vi "ANAL_DeriveData.vi"(10 "GUI Cluster":T1, 11 "Main Data Array":T2 {"Run Data Cluster"."Temperature B" scale=0.0..100.0; "Run Data Cluster"."Temperature A" scale=0.0..100.0}) -> (2 "GUI Cluster Out":T1, 3 "Main Data Array Out":T2 {"Run Data Cluster"."Temperature B" scale=0.0..100.0; "Run Data Cluster"."Temperature A" scale=0.0..100.0})   [LabVIEW 2021]
uses:
  ANAL_Data.ctl
  XML_Cluster.ctl
  DAT_Cluster.ctl
  ANAL_GUIStatus.ctl
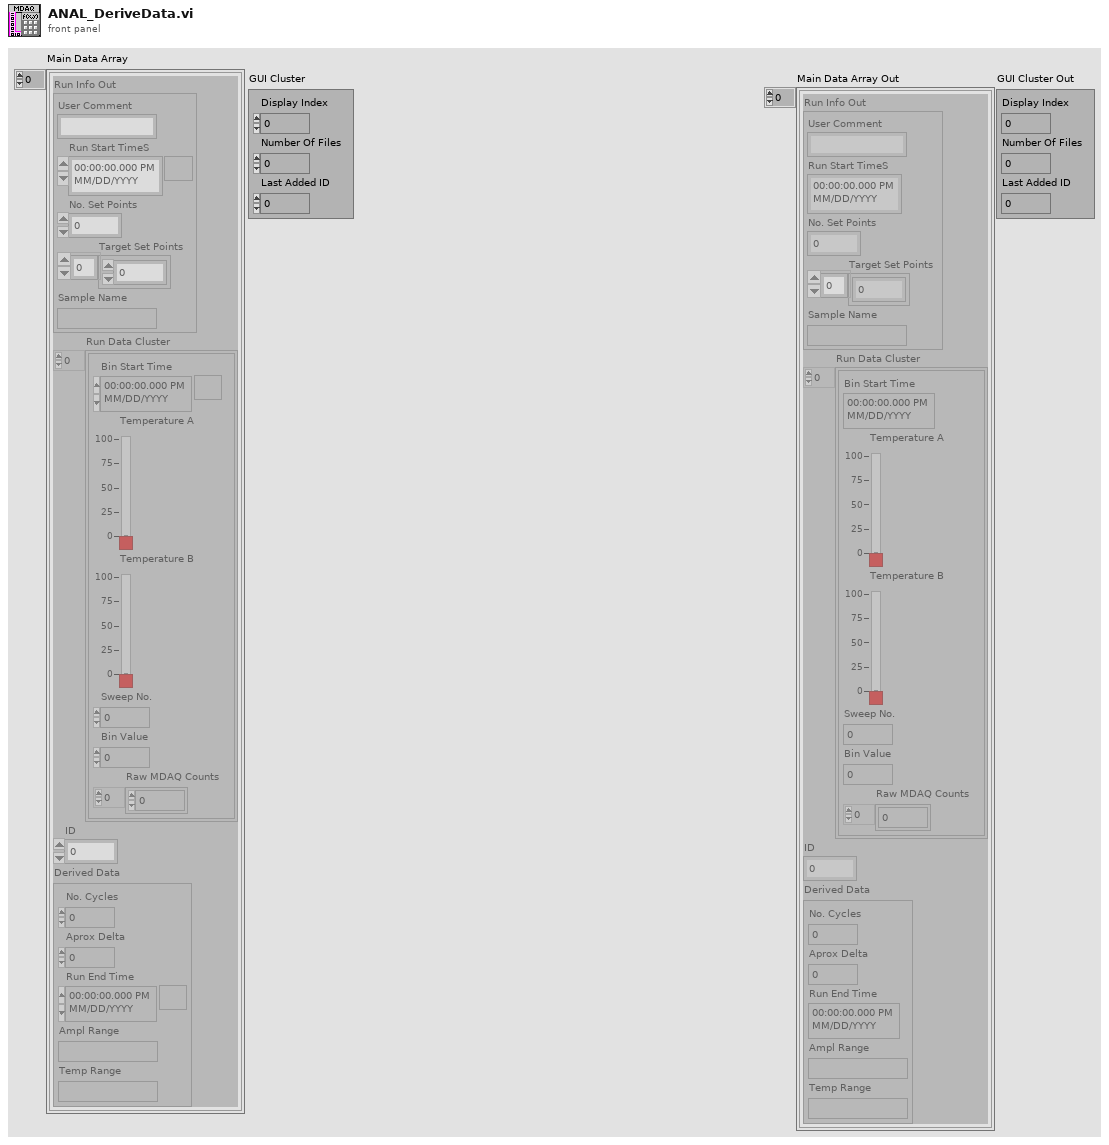
[diagram p1: front panel]
types:
  T1 = typedef "ANAL_GUIStatus.ctl" = cluster{"Display Index":i32, "Number Of Files":u32, "Last Added ID":u32}
  T2 = typedef "ANAL_Data.ctl" = cluster{"Run Info Out":T3, "Run Data Cluster":T4, "ID":u32, "Derived Data":cluster{"No. Cycles":u32, "Aprox Delta":dbl, "Run End Time":timestamp, "Ampl Range":string, "Temp Range":string}}[]
  T3 = typedef "XML_Cluster.ctl" = cluster{"User Comment":string, "Run Start TimeS":timestamp, "No. Set Points":u32, "Target Set Points":i32[], "Sample Name":string}
  T4 = typedef "DAT_Cluster.ctl" = cluster{"Bin Start Time":timestamp, "Temperature A":dbl, "Temperature B":dbl, "Sweep No.":i32, "Bin Value":i32, "Raw MDAQ Counts":i32[]}[]
  T5 = cluster{"Run Info Out":T3, "Run Data Cluster":T4, "ID":u32, "Derived Data":cluster{"No. Cycles":u32, "Aprox Delta":dbl, "Run End Time":timestamp, "Ampl Range":string, "Temp Range":string}}
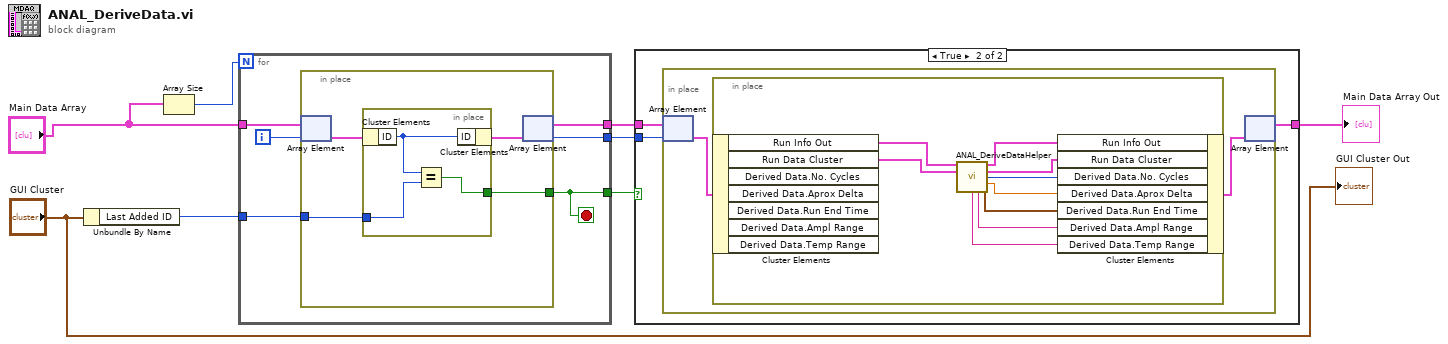
[diagram p0: block diagram]
diagram:
  n1 = Unbundle By Name("GUI Cluster") -> ("Last Added ID"=w8:u32)
  n2 = Array Size(array="Main Data Array") -> (size(s)=w6:i32)
  n3 = for {
    N: w6 -> [_]
    tunnel: "Main Data Array" -> [w14]
    tunnel: w8 -> [w12]
    tunnel: [w11] -> w3
    tunnel: [w10] -> w4
    tunnel: [w9] -> w5
    i -> [w13]
    stop <- w9 stop-if-true
    n4 = in-place {
      in-place-border: w12 -> [w17]
      in-place-border: [w16] -> w9
      n5 = in-place-array #1(w14, w13) -> (w18:T5)
      n6 = in-place {
        in-place-border: w17 -> [w21]
        in-place-border: [w19] -> w16
        n7 = in-place-cluster #2(w18) -> ("ID"=w20:u32)
        n8 = Equal?(x=w20, y=w21) -> (x = y?=w19:bool)
        n9 = in-place-cluster #2("ID"=w20) -> (w15:T5)
      }
      n10 = in-place-array #1(w15) -> (w10:T2, w11:i32)
    }
  }
  n11 = case shown="True" w5 {
    tunnel: w4 -> [w22 w25]
    tunnel: w3 -> [_ w24]
    tunnel: [w22 w23] -> w2
    frame False {
    }
    frame True {
      n12 = in-place {
        n13 = in-place-array #3(w25, w24) -> (w27:T5)
        n14 = in-place {
          n15 = in-place-cluster #4(w27) -> ("Run Info Out"=w36:T3, "Run Data Cluster"=w35:T4)  [unwired: 5 out]
          n16 = call "ANAL_DeriveDataHelper.vi"("Run Info Out"=w36, "Run Data Cluster"=w35) -> ("Run Info Out 2"=w34:T3, "Run Data Cluster 2"=w33:T4, "No. Sweeps"=w32:i32, "Delta"=w31:dbl, "Temp Range"=w28:string, "Ampl Range"=w29:string, "End Time"=w30:timestamp)  [unwired: 7 in]
          n17 = in-place-cluster #4("Run Info Out"=w34, "Run Data Cluster"=w33, "Derived Data.No. Cycles"=w32, "Derived Data.Aprox Delta"=w31, "Derived Data.Run End Time"=w30, "Derived Data.Ampl Range"=w29, "Derived Data.Temp Range"=w28) -> (w26:T5)
        }
        n18 = in-place-array #3(w26) -> (w23:T2)  [unwired: 1 out]
      }
    }
  }
  "Main Data Array Out" <- w2
  "GUI Cluster Out" <- "GUI Cluster"
